vi "Set Z-ROI.vi"(8 "error in":errorcluster, 10 "Z - ROI":cluster{"Index":u32, "Length":u32}, 11 "Graph with Analysis Controls in":refnum<class "Graph with Analysis Controls.lvclass">) -> (0 "error out":errorcluster, 3 "Graph with Analysis Controls out":refnum<class "Graph with Analysis Controls.lvclass">)   [LabVIEW 2023, in "Graph with Analysis Controls.lvclass"]
uses:
  Graph with Analysis Controls.lvclass
  Graph with Analysis Controls.lvclass/Graph with Analysis Controls.ctl
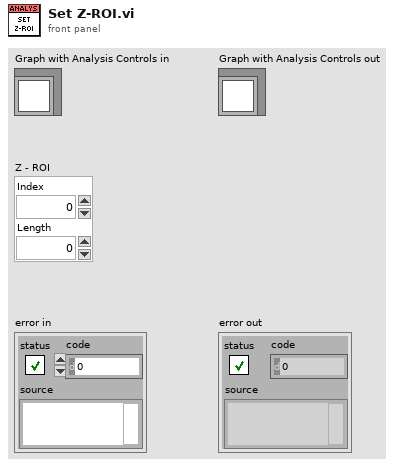
[diagram p1: front panel]
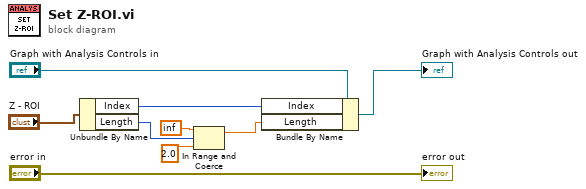
[diagram p0: block diagram]
diagram:
  n1 = Unbundle By Name("Z - ROI") -> ("Index"=w5:u32, "Length"=w4:u32)
  n2 = In Range and Coerce(upper limit=inf, x=w4, lower limit=2.0) -> (coerced(x)=w1:dbl)  [unwired: 1 out]
  n3 = Bundle By Name(cluster="Graph with Analysis Controls in", "Index"=w5, "Length"=w1) -> (→"Graph with Analysis Controls out":refnum<class "Graph with Analysis Controls.lvclass">)
  "error out" <- "error in"
